vi "pressKey2020.vi"(8 "time":dbl, 9 "Virtual Key":u8(ring)=65) -> ()   [LabVIEW 2020]
doc: "call keybd_event drom user32.dll library to generate the key down event on desired key"
uses:
  user32.dll
panel:
  # "Key press subVI"
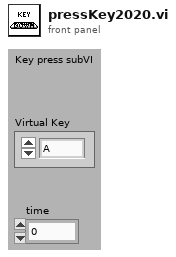
[diagram p1: front panel]
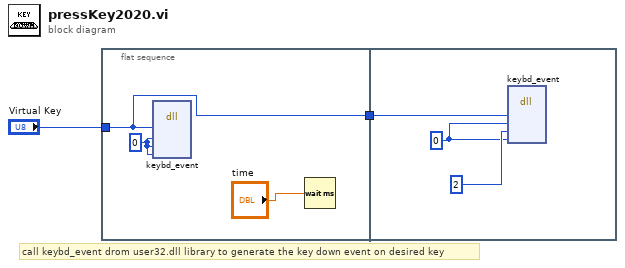
[diagram p0: block diagram]
diagram:
  # "call keybd_event drom user32.dll library to generate the key down event on desired key"
  n1 = flat-sequence {
    tunnel: "Virtual Key" -> [w4]
    tunnel: [w4] -> w2
    tunnel: w2 -> [w8]
    frame #0 {
      w5 = u8 0 ("bScan")
      n2 = dll-call lib="user32.dll" fn="keybd_event"("bVk"=w4, "bScan"=w5, "dwFlags"=w5, "dwExtraInfo"=w5) -> ()  [unwired: 8 in, 2 out]
      n3 = Wait (ms)(milliseconds to wait="time") -> ()  [unwired: 1 out]
    }
    frame #1 {
      w6 = 0
      n4 = dll-call lib="user32.dll" fn="keybd_event"("bVk"=w8, "bScan"=w6, "dwFlags"=2, "dwExtraInfo"=w6) -> ()  [unwired: 8 in, 2 out]
    }
  }
